vi "Reset stop flag.vi"(8 "error in (no error)":errorcluster) -> (0 "error out":errorcluster)   [LabVIEW 2020, in "core.lvlib"]
uses:
  core.lvlib
  stop_core (global variable).vi
panel:
  # "Development\ncontrols/indicators useful for development and testing, but which are not outputs of the VI"
  # "Input\nInputs to the VI"
  # "Output\nOutputs of the VI"
  # "Description\n\nBlank VI with error handling case. \n\nSummarize the use of this VI in this space."
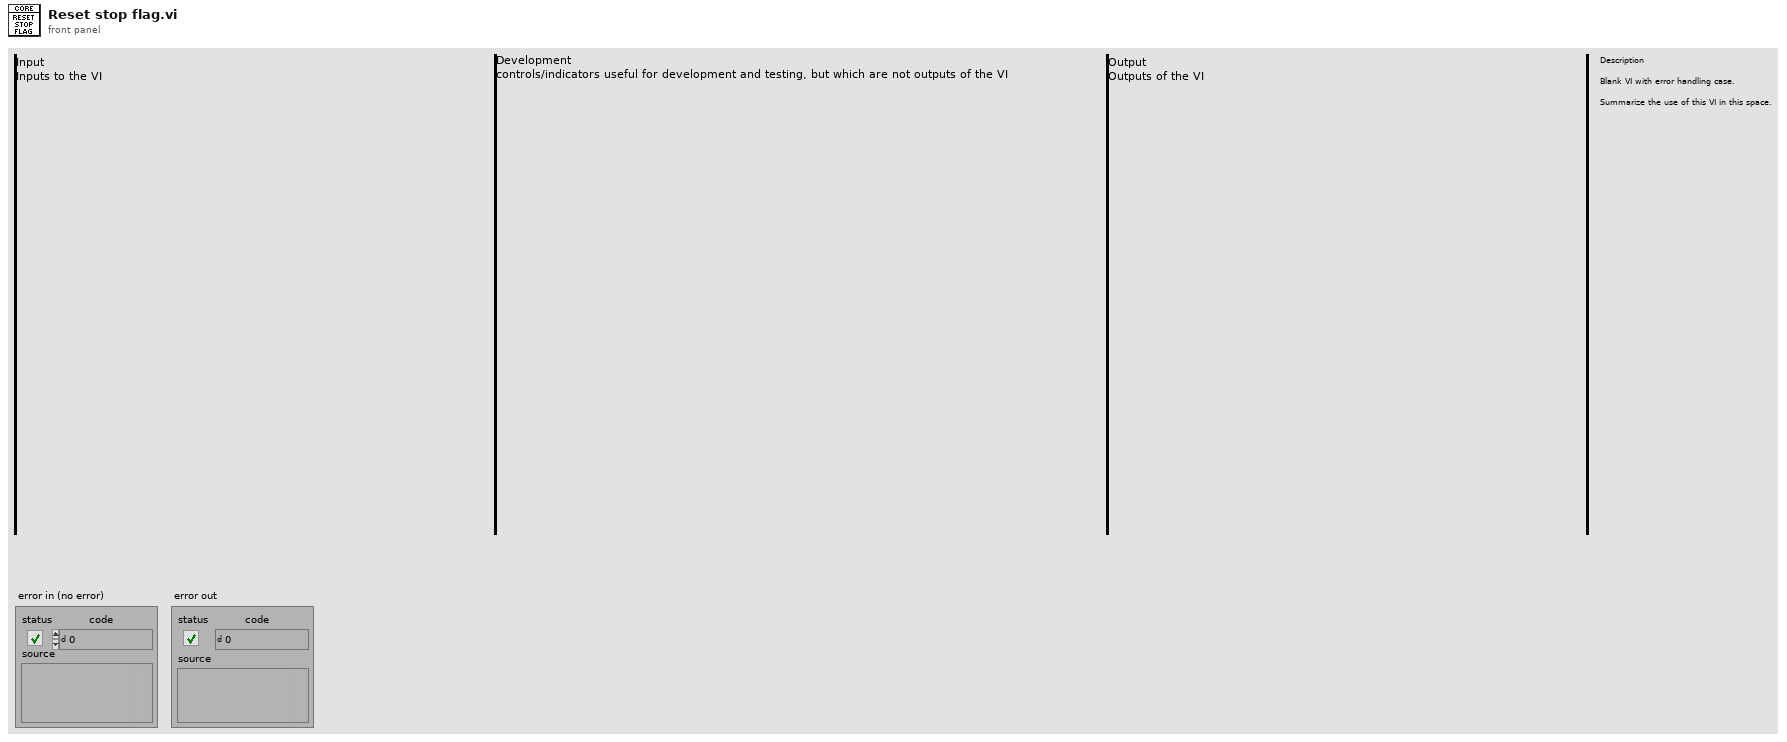
[diagram p1: front panel]
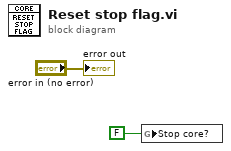
[diagram p0: block diagram]
diagram:
  n1 = global write "stop_core (global variable).vi" "Stop core?"(FALSE ("Stop core?")) -> ()
  "error out" <- "error in (no error)"
